vi "Teleop.vi"(10 "Match Info":T1={"Autonomous Elapsed Seconds"=0.0, "TeleOp Elapsed Seconds"=0.0, "Disabled Elapsed Seconds"=0.0, "Visited Autonomous"=FALSE, "Visited TeleOp"=FALSE, "Visited Disabled"=FALSE, "Autonomous Settings"={"Autonomous Style"=enum."Independent", "VI Refnum"=refnum}}, 11 "Call Context":T2) -> ()   [LabVIEW 2013]
doc: "This VI is called for each TeleOp packet received from the DS where the robot is not disabled. It is often used to read from the joysticks and update I/O or to update setpoints for timed control loops. It should complete and return within 20 milliseconds or it may miss DS packets."
uses:
  <vilib>/Rock Robotics/WPI/DriverStation/WPI_DriverStationDerivedRobotMode.ctl
  <vilib>/Rock Robotics/WPI/DriverStation/WPI_DriverStationMatch Info.ctl
  Robot Global Data.vi
  <vilib>/Rock Robotics/WPI/Joystick/WPI_JoystickGetSetRefNum.vi
panel:
  in  "Left":bool
  in  "Right":bool
  in  "Shifter":bool
  in  "HarvSpeed":dbl=0.5
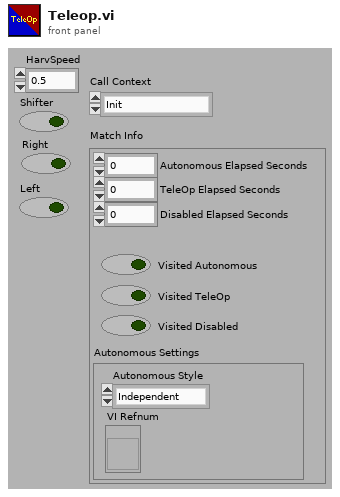
[diagram p1: front panel]
types:
  T1 = typedef "WPI_DriverStationMatch Info.ctl" = cluster{"Autonomous Elapsed Seconds":dbl, "TeleOp Elapsed Seconds":dbl, "Disabled Elapsed Seconds":dbl, "Visited Autonomous":bool, "Visited TeleOp":bool, "Visited Disabled":bool, "Autonomous Settings":cluster{"Autonomous Style":enum16{"Iterative", "Independent"}, "VI Refnum":refnum<vi>}}
  T2 = typedef "WPI_DriverStationDerivedRobotMode.ctl" = enum16{"Init", "Execute", "Stop"}
  T3 = typedef "WPI_JoystickDevRef.ctl" = cluster{"Device":T4}
  T4 = typedef "WPI_JoystickDeviceEnum.ctl" = enum16{"USB 1", "USB 2", "USB 3", "USB 4", "Kinect 1", "Kinect 2"}
  T5 = cluster{"axis 1 (x)":dbl, "axis 2 (y)":dbl, "axis 3 (throttle)":dbl, "axis 4":dbl, "axis 5":dbl, "axis 6":dbl}
  T6 = typedef "WPI_MotorControlDeviceRef.ctl" = cluster{"DeviceStatus":errorcluster, "Type":enum16{"PWM", "CAN"}, "PWM":cluster{"Digital Module":T7, "PWM Channel":T8, "DeadBand":T9}, "CAN":cluster{"Device Number":u8, "Control Mode":T10, "Semaphore":T11, "Max Vout":dbl}, "Invert":bool, "TransformRef":T12, "InvTransformRef":T12}
  T7 = typedef "FPGA_TypedefDigitalModule.ctl" = enum16{"Digital Module 1", "Digital Module 2"}
  T8 = typedef "FPGA_DIOPWMChannel.ctl" = enum8{"PWM 1", "PWM 2", "PWM 3", "PWM 4", "PWM 5", "PWM 6", "PWM 7", "PWM 8", "PWM 9", "PWM 10", "Invalid"}
  T9 = typedef "WPI_PWMDeadband.ctl" = cluster{"Name":string, "maxPositivePwm":i32, "minPositivePwm":i32, "centerPwm":i32, "maxNegativePwm":i32, "minNegativePwm":i32, "angularRange":u16}
  T10 = typedef "WPI_CANJaguar_ControlMode.ctl" = enum8{"Percent VBus", "Current", "Speed", "Position", "Voltage"}
  T11 = typedef "Semaphore RefNum" = refnum<k1>
  T12 = typedef "WPI_PWMTransform_ConPane.ctl" = refnum<vi>
  T13 = cluster{"Driver Station Digital Input (1-8)[0]":bool, "Driver Station Digital Input (1-8)[1]":bool, "Driver Station Digital Input (1-8)[2]":bool, "Driver Station Digital Input (1-8)[3]":bool, "Driver Station Digital Input (1-8)[4]":bool, "Driver Station Digital Input (1-8)[5]":bool, "Driver Station Digital Input (1-8)[6]":bool, "Driver Station Digital Input (1-8)[7]":bool, "Driver Station Digital Input (1-8)[8]":bool}
  T14 = cluster{"RightLow":dbl, "LeftLow":dbl, "RightHigh":dbl, "LeftHigh":dbl}
  T15 = typedef "WPI_JoystickButtonState.ctl" = cluster{"Button 1":bool, "Button 2":bool, "Button 3":bool, "Button 4":bool, "Button 5":bool, "Button 6":bool, "Button 7":bool, "Button 8":bool, "Button 9":bool, "Button 10":bool, "Button 11":bool, "Button 12":bool}
  T16 = typedef "WPI_ServoDeviceRef.ctl" = cluster{"DeviceStatus":errorcluster, "Digital Module":T7, "PWM Channel":T8, "DeadBand":T9}
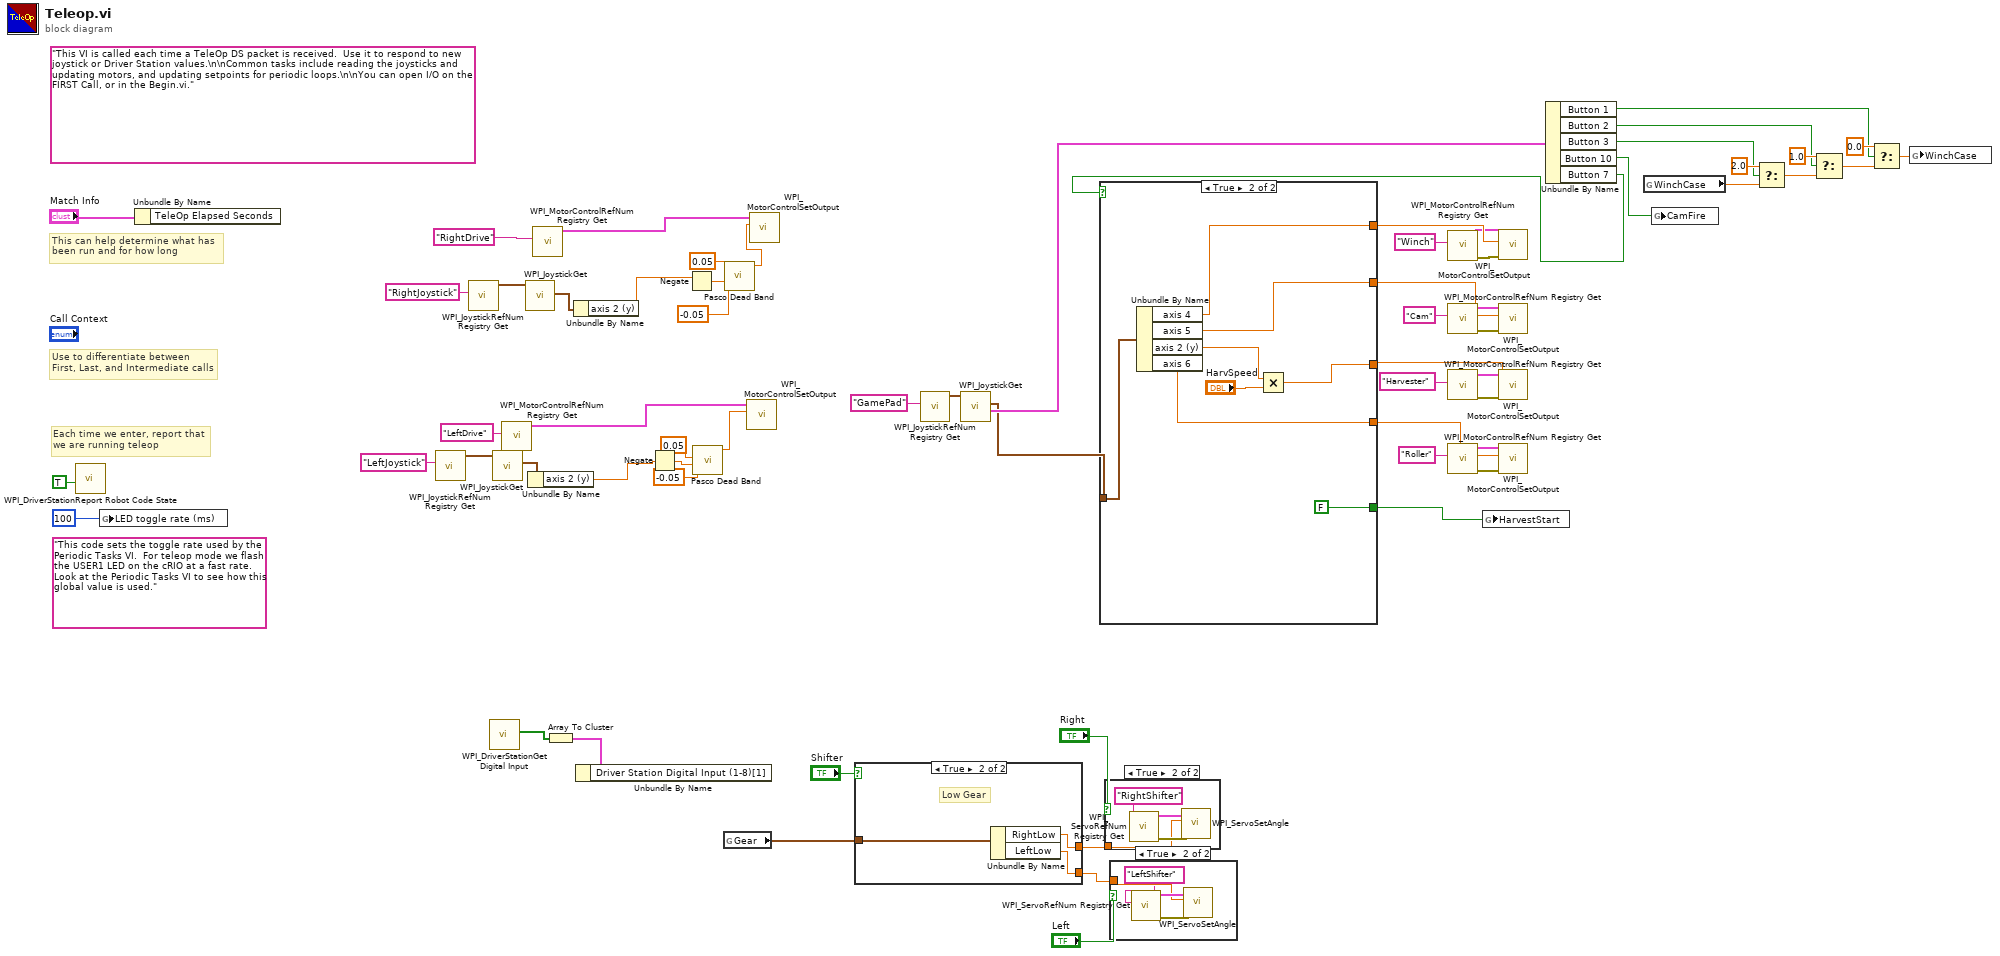
[diagram p0: block diagram]
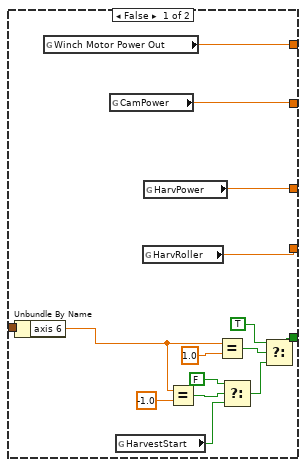
[diagram p2: hidden frame]
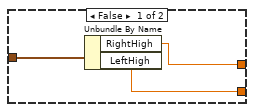
[diagram p4: hidden frame]
diagram:
  (unwired) "This code sets the toggle rate used by the Periodic Tasks VI.  For teleop mode we flash the USER1 LED on the cRIO at a fast rate.  Look at the Periodic Tasks VI to see how this global value is used."
  (unwired) "This VI is called each time a TeleOp DS packet is received.  Use it to respond to new joystick or Driver Station values.\n\nCommon tasks include reading the joysticks and updating motors, and updating setpoints for periodic loops.\n\nYou can open I/O on the FIRST Call, or in the Begin.vi."
  # "Each time we enter, report that\nwe are running teleop"
  # "Use to differentiate between\nFirst, Last, and Intermediate calls"
  # "This can help determine what has\nbeen run and for how long"
  n1 = call <vilib>:"WPI_DriverStationReport Robot Code State.vi"("TeleOp"=TRUE ("Autonomous")) -> ()  [unwired: 10 in, 1 out]
  n2 = global write "Robot Global Data.vi" "LED toggle rate (ms)"(u32 100 ("LED ms toggle rate")) -> ()
  n3 = Unbundle By Name("Match Info") -> ()  [unwired: 1 out]
  n4 = call <vilib>:"WPI_JoystickRefNum Registry Get.vi"("refnum name"="LeftJoystick") -> ("JoystickDevRef"=w53:T3)  [unwired: 9 in, 1 out]
  n5 = call <vilib>:"WPI_JoystickRefNum Registry Get.vi"("refnum name"="RightJoystick") -> ("JoystickDevRef"=w58:T3)  [unwired: 9 in, 1 out]
  n6 = call <vilib>:"WPI_DriverStationGet Digital Input.vi"() -> ("Driver Station Digital Input (1-8)"=w41:bool[])  [unwired: 11 in]
  n7 = call <vilib>:"WPI_JoystickGet.vi"("JoystickDevRef"=w53) -> ("Axes"=w52:T5)  [unwired: 4 in, 2 out]
  n8 = call <vilib>:"WPI_MotorControlRefNum Registry Get.vi"("refnum name"="LeftDrive") -> ("MotorControlDevRef"=w56:T6)  [unwired: 9 in, 1 out]
  n9 = call <vilib>:"WPI_JoystickGet.vi"("JoystickDevRef"=w58) -> ("Axes"=w57:T5)  [unwired: 4 in, 2 out]
  n10 = Unbundle By Name(w52) -> ("axis 2 (y)"=w51:dbl)
  n11 = call <vilib>:"WPI_MotorControlRefNum Registry Get.vi"("refnum name"="RightDrive") -> ("MotorControlDevRef"=w61:T6)  [unwired: 9 in, 1 out]
  n12 = Array To Cluster(array=w41) -> (cluster=w40:T13)
  n13 = Unbundle By Name(w57) -> ("axis 2 (y)"=w50:dbl)
  n14 = Unbundle By Name(w40) -> ()  [unwired: 1 out]
  n15 = Negate(x=w51) -> (-x=w45:dbl)
  n16 = Negate(x=w50) -> (-x=w49:dbl)
  n17 = call "Pasco Dead Band.vi"("lower limit"=-0.05, "PWM Power"=w45, "upper limit"=0.05) -> ("PWM Power"=w42:dbl)  [unwired: 7 in, 1 out]
  n18 = global read "Robot Global Data.vi" "Gear"() -> (w39:T14)
  n19 = call "Pasco Dead Band.vi"("lower limit"=-0.05, "PWM Power"=w49, "upper limit"=0.05) -> ("PWM Power"=w48:dbl)  [unwired: 7 in, 1 out]
  n20 = call <vilib>:"WPI_MotorControlSetOutput.vi"("Output"=w42, "MotorControlDevRef"=w56) -> ()  [unwired: 7 in, 3 out]
  n21 = call <vilib>:"WPI_MotorControlSetOutput.vi"("Output"=w48, "MotorControlDevRef"=w61) -> ()  [unwired: 7 in, 3 out]
  n22 = case shown="True" "Shifter" {
    tunnel: w39 -> [w67 w70]
    tunnel: [w66 w69] -> w38
    tunnel: [w65 w68] -> w37
    frame False {
      n23 = Unbundle By Name(w67) -> ("RightHigh"=w66:dbl, "LeftHigh"=w65:dbl)
    }
    frame True {
      # "Low Gear"
      n24 = Unbundle By Name(w70) -> ("RightLow"=w69:dbl, "LeftLow"=w68:dbl)
    }
  }
  n25 = call <vilib>:"WPI_JoystickRefNum Registry Get.vi"("refnum name"="GamePad") -> ("JoystickDevRef"=w32:T3)  [unwired: 9 in, 1 out]
  n26 = call <vilib>:"WPI_JoystickGet.vi"("JoystickDevRef"=w32) -> ("Buttons"=w5:T15, "Axes"=w3:T5)  [unwired: 4 in, 1 out]
  n27 = case shown="True" "Right" {
    tunnel: w38 -> [_ w71]
    frame False {
    }
    frame True {
      n28 = call <vilib>:"WPI_ServoRefNum Registry Get.vi"("refnum name"="RightShifter") -> ("error out"=w74:errorcluster, "ServoDeviceRef"=w73:T16)  [unwired: 9 in]
      n29 = call <vilib>:"WPI_ServoSetAngle.vi"("error in (no error)"=w74, "Angle"=w71, "ServoDeviceRef"=w73) -> ()  [unwired: 7 in, 2 out]
    }
  }
  n30 = case shown="True" "Left" {
    tunnel: w37 -> [_ w76]
    frame False {
    }
    frame True {
      n31 = call <vilib>:"WPI_ServoRefNum Registry Get.vi"("refnum name"="LeftShifter") -> ("error out"=w77:errorcluster, "ServoDeviceRef"=w78:T16)  [unwired: 9 in]
      n32 = call <vilib>:"WPI_ServoSetAngle.vi"("error in (no error)"=w77, "Angle"=w76, "ServoDeviceRef"=w78) -> ()  [unwired: 7 in, 2 out]
    }
  }
  n33 = call <vilib>:"WPI_MotorControlRefNum Registry Get.vi"("refnum name"="Winch") -> ("error out"=w23:errorcluster, "MotorControlDevRef"=w17:T6)  [unwired: 9 in]
  n34 = call <vilib>:"WPI_MotorControlRefNum Registry Get.vi"("refnum name"="Cam") -> ("error out"=w22:errorcluster, "MotorControlDevRef"=w21:T6)  [unwired: 9 in]
  n35 = call <vilib>:"WPI_MotorControlRefNum Registry Get.vi"("refnum name"="Harvester") -> ("error out"=w27:errorcluster, "MotorControlDevRef"=w26:T6)  [unwired: 9 in]
  n36 = call <vilib>:"WPI_MotorControlRefNum Registry Get.vi"("refnum name"="Roller") -> ("error out"=w29:errorcluster, "MotorControlDevRef"=w30:T6)  [unwired: 9 in]
  n37 = Unbundle By Name(w5) -> ("Button 1"=w8:bool, "Button 2"=w9:bool, "Button 3"=w10:bool, "Button 10"=w4:bool, "Button 7"=w1:bool)
  n38 = case shown="True" w1 {
    tunnel: [w93 w100] -> w28
    tunnel: [w92 w95] -> w24
    tunnel: w3 -> [w80 w101]
    tunnel: [w90 w99] -> w18
    tunnel: [w91 w98] -> w16
    tunnel: [w79 FALSE ("HarvestStart")] -> w2
    frame False {
      n39 = Unbundle By Name(w80) -> ("axis 6"=w88:dbl)
      n40 = global read "Robot Global Data.vi" "Winch Motor Power Out"() -> (w90:dbl)
      n41 = global read "Robot Global Data.vi" "CamPower"() -> (w91:dbl)
      n42 = global read "Robot Global Data.vi" "HarvestStart"() -> (w89:bool)
      n43 = global read "Robot Global Data.vi" "HarvRoller"() -> (w93:dbl)
      n44 = global read "Robot Global Data.vi" "HarvPower"() -> (w92:dbl)
      n45 = Equal?(x=w88, y=-1.0) -> (x = y?=w87:bool)
      n46 = Equal?(x=w88, y=1.0) -> (x = y?=w82:bool)
      n47 = Select(t=FALSE, s=w87, f=w89) -> (s? t:f=w85:bool)
      n48 = Select(t=TRUE, s=w82, f=w85) -> (s? t:f=w79:bool)
    }
    frame True {
      n49 = Unbundle By Name(w101) -> ("axis 4"=w99:dbl, "axis 5"=w98:dbl, "axis 2 (y)"=w96:dbl, "axis 6"=w100:dbl)
      n50 = Multiply(x=w96, y="HarvSpeed") -> (x*y=w95:dbl)
    }
  }
  n51 = global write "Robot Global Data.vi" "HarvestStart"(w2) -> ()
  n52 = call <vilib>:"WPI_MotorControlSetOutput.vi"("error in (no error)"=w23, "Output"=w18, "MotorControlDevRef"=w17) -> ()  [unwired: 6 in, 3 out]
  n53 = call <vilib>:"WPI_MotorControlSetOutput.vi"("error in (no error)"=w22, "Output"=w16, "MotorControlDevRef"=w21) -> ()  [unwired: 6 in, 3 out]
  n54 = call <vilib>:"WPI_MotorControlSetOutput.vi"("error in (no error)"=w27, "Output"=w24, "MotorControlDevRef"=w26) -> ()  [unwired: 6 in, 3 out]
  n55 = call <vilib>:"WPI_MotorControlSetOutput.vi"("error in (no error)"=w29, "Output"=w28, "MotorControlDevRef"=w30) -> ()  [unwired: 6 in, 3 out]
  n56 = global read "Robot Global Data.vi" "WinchCase"() -> (w6:dbl)
  n57 = global write "Robot Global Data.vi" "CamFire"(w4) -> ()
  n58 = Select(t=2.0, s=w10, f=w6) -> (s? t:f=w15:dbl)
  n59 = Select(t=1.0, s=w9, f=w15) -> (s? t:f=w14:dbl)
  n60 = Select(t=0.0, s=w8, f=w14) -> (s? t:f=w7:dbl)
  n61 = global write "Robot Global Data.vi" "WinchCase"(w7) -> ()
